vi "GetRefByLabel.vi"(7 "InsideTab":bool, 8 "error in":errorcluster, 11 "Label":string) -> (0 "error out":errorcluster, 1 "Encontrado?":bool, 3 "Ctl Refnum":refnum<vi>)   [LabVIEW 2018]
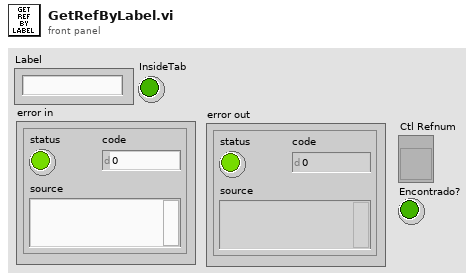
[diagram p1: front panel]
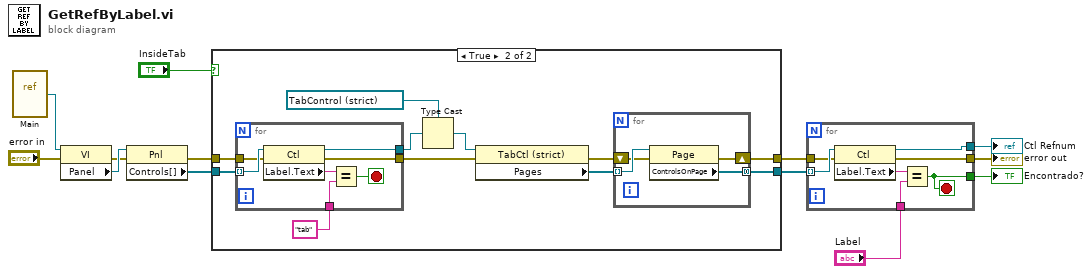
[diagram p0: block diagram]
diagram:
  n1 = vi-ref "Main.vi"() -> (w13:refnum<vi>)
  n2 = property class="VI"(reference=w13, error in="error in") -> (error out=w8:errorcluster, "Panel"=w12:refnum<vi>)  [unwired: 1 out]
  n3 = property class="Pnl"(reference=w12, error in=w8) -> (error out=w4:errorcluster, "Controls[]"=w2:refnum<vi>[])  [unwired: 1 out]
  n4 = case shown="True" "InsideTab" {
    tunnel: w4 -> [w15 w26]
    tunnel: [w15 w16] -> w3
    tunnel: w2 -> [w14 w25]
    tunnel: [w14 w17] -> w1
    frame False {
    }
    frame True {
      n5 = for {
        tunnel: w25 -> [w37] mode=indexing
        tunnel: "tab" ("Label") -> [w35]
        tunnel: [w34] -> w23
        tunnel: w26 -> [w33]
        tunnel: [w32] -> w20
        stop <- w31 stop-if-true
        n6 = property class="Ctl"(reference=w37, error in=w33) -> (reference out=w34:refnum<vi>, error out=w32:errorcluster, "Label.Text"=w36:string)
        n7 = Equal?(x=w36, y=w35) -> (x = y?=w31:bool)
      }
      n8 = Type Cast(type=refnum<vi> refnum ("tab"), x=w23) -> (*(type *) &x=w21:refnum<vi>)
      n9 = property class="TabCtl (strict)"(reference=w21, error in=w20) -> (error out=w18:errorcluster, "Pages"=w19:refnum<vi>[])  [unwired: 1 out]
      n10 = for {
        tunnel: w19 -> [w30] mode=indexing
        shift-right: [w27] -> w16
        shift-left: w18 -> [w29]
        tunnel: [w28] -> w17 mode=concatenating
        n11 = property class="Page"(reference=w30, error in=w29) -> (error out=w27:errorcluster, "ControlsOnPage"=w28:refnum<vi>[])  [unwired: 1 out]
      }
    }
  }
  n12 = for {
    tunnel: w1 -> [w44] mode=indexing
    tunnel: "Label" -> [w42]
    tunnel: [w41] -> w10
    tunnel: w3 -> [w40]
    tunnel: [w39] -> w7
    tunnel: [w38] -> w6
    stop <- w38 stop-if-true
    n13 = property class="Ctl"(reference=w44, error in=w40) -> (reference out=w41:refnum<vi>, error out=w39:errorcluster, "Label.Text"=w43:string)
    n14 = Equal?(x=w43, y=w42) -> (x = y?=w38:bool)
  }
  "Ctl Refnum" <- w10
  "error out" <- w7
  "Encontrado?" <- w6
